vi "Process.vi"(8 "error in":errorcluster, 11 "Instrument":refnum<class "Instrument.lvclass">) -> (0 "error out":errorcluster, 3 "Instrument out":refnum<class "Instrument.lvclass">)   [LabVIEW 2019, in "Instrument.lvlib" / "Instrument.lvclass"]
doc: "---------------------------------------------------------------\nJKI State Machine Objects™\nhttp://jki.net/state-machine-objects/\nCopyright (C) 2005-2015, JKI <info@jki.net>\nALL RIGHTS RESERVED"
uses:
  Instrument.lvclass
  C:/Program Files/National Instruments/LabVIEW 2019/vi.lib/JKI/JKI SMO/SMO/SMO.lvclass
  <userlib>/LevyLab/RemoteControl/RemoteControl/Typedefs/Message--Cluster.ctl
  <vilib>/JKI/JKI SMO/SMO/SMO.lvclass/SMO.ctl
  <vilib>/dlg_ctls.llb/Space Constant.vi
  <vilib>/AdvancedString/1D String Array to Delimited String.vi
  <vilib>/JKI/JKI SMO/SMO/Private/ReftoDVR--SMO.vi
  <userlib>/LevyLab/RemoteControl/RemoteControl/RemoteControl.lvclass
  <userlib>/LevyLab/Logger.Error/Logger.Error/Logger.Error.lvclass
  <userlib>/LevyLab/Logger.PGSQL/Logger.PGSQL/Logger.PGSQL.lvclass
  <vilib>/JKI/JKI SMO/SMO/SMO.lvclass
  <userlib>/LevyLab/Debug/Debug.lvlib
panel:
  out "State History":string
  out "Name":string
  out "Command":string
  # "1. Receives & processes commands from RemoteControl process\n2. Logs instrument settings to PGSQL using Logger process"
  # "INSTRUMENT"
  # "INSTRUMENT"
  # "For instructions on how to use the JKI State Machine Objects, examples and video tutorials, visit:\nhttp://jki.net/state-machine-objects/\n\nJKI State Machine Objects™\nhttp://jki.net/state-machine-objects/\nCopyright (C) 2005-2015, JKI <info@jki.net>\nALL RIGHTS RESERVED"
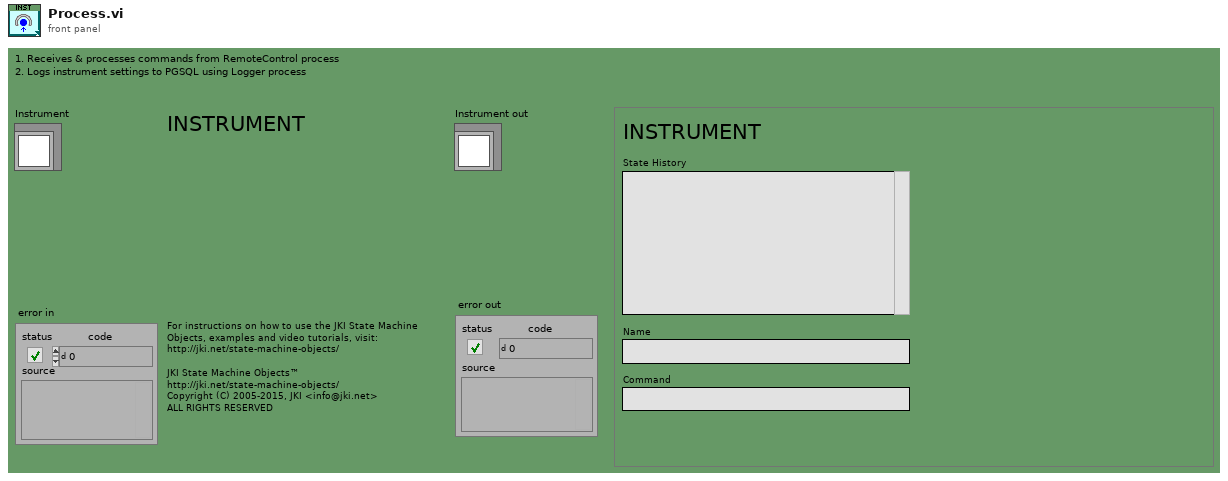
[diagram p1: front panel]
types:
  T1 = enum32{"invalid app kind", "Development System", "Run Time System", "Student Edition", "Embedded LabVIEW", "Evaluation", "Custom"}
  T2 = enum32{"Invalid", "Standard", "Closed", "Hidden", "Minimized", "Maximized"}
  T3 = typedef "RemoteControl.lvlib/RemoteControl.lvclass/Message--Cluster.ctl" = cluster{"Command":string, "Data":variant, "ID":string}
  T4 = typedef "Instrument.lvlib/Instrument.lvclass/Dependencies--Cluster.ctl" = cluster{"API":refnum<class "API.lvclass">, "Configuration":refnum<class "Configuration.lvclass">, "HAL":refnum<class "HAL.lvclass">, "DB-Logger":refnum<class "Logger.PGSQL.lvclass">, "Error-Logger":refnum<class "Logger.Error.lvclass">, "Remote-Control":refnum<class "RemoteControl.lvclass">}
  T5 = cluster{"Core":cluster{"Current VI Reference":refnum<vi>, "Close Panel on Exit?":bool, "Last Error":cluster{"error":errorcluster, "previous state":string, "remaining states":string}, "Shutdown?":bool}, "SelfRef":refnum<class "Instrument.lvclass">, "Dependencies":T4, "Message":T3}
  T6 = typedef "RemoteControl.lvclass/Message--Cluster.ctl" = cluster{"Command":string, "Data":variant, "ID":string}
  T7 = typedef "SMO.lvclass/SMOState --Enum.ctl" = enum16{"unknown", "Created", "Started", "Stopped"}
  T8 = cluster{"Current VI Reference":refnum<vi>, "Close Panel on Exit?":bool, "Last Error":cluster{"error":errorcluster, "previous state":string, "remaining states":string}, "Shutdown?":bool}
  T9 = typedef "Debug.lvlib/Attribute.Debug.lvclass/DebugBehavior.ctl" = enum16{"Normal", "Debug"}
  T10 = typedef "SMO.lvclass/Protected Events.ctl" = cluster{"StopProcesses":refnum<user-event>, "AbortProcesses":refnum<user-event>, "Config Changed":refnum<user-event>, "Dependency":refnum<user-event>}
  T11 = typedef "Instrument.lvlib/Instrument.lvclass/PrivateEvents--Cluster.ctl" = cluster{"MessageToProcess":refnum<user-event>, "LogData":refnum<user-event>, "LogDataMultiline":refnum<user-event>}
  T12 = typedef "RemoteControl.lvlib/RemoteControl.lvclass/PublicEvents--Cluster.ctl" = cluster{"SendMessageFromProcess":refnum<user-event>}
  T13 = typedef "SMO.lvclass/Public Events.ctl" = cluster{"Error":refnum<user-event>, "State":refnum<user-event>, "Reserve State":refnum<user-event>}
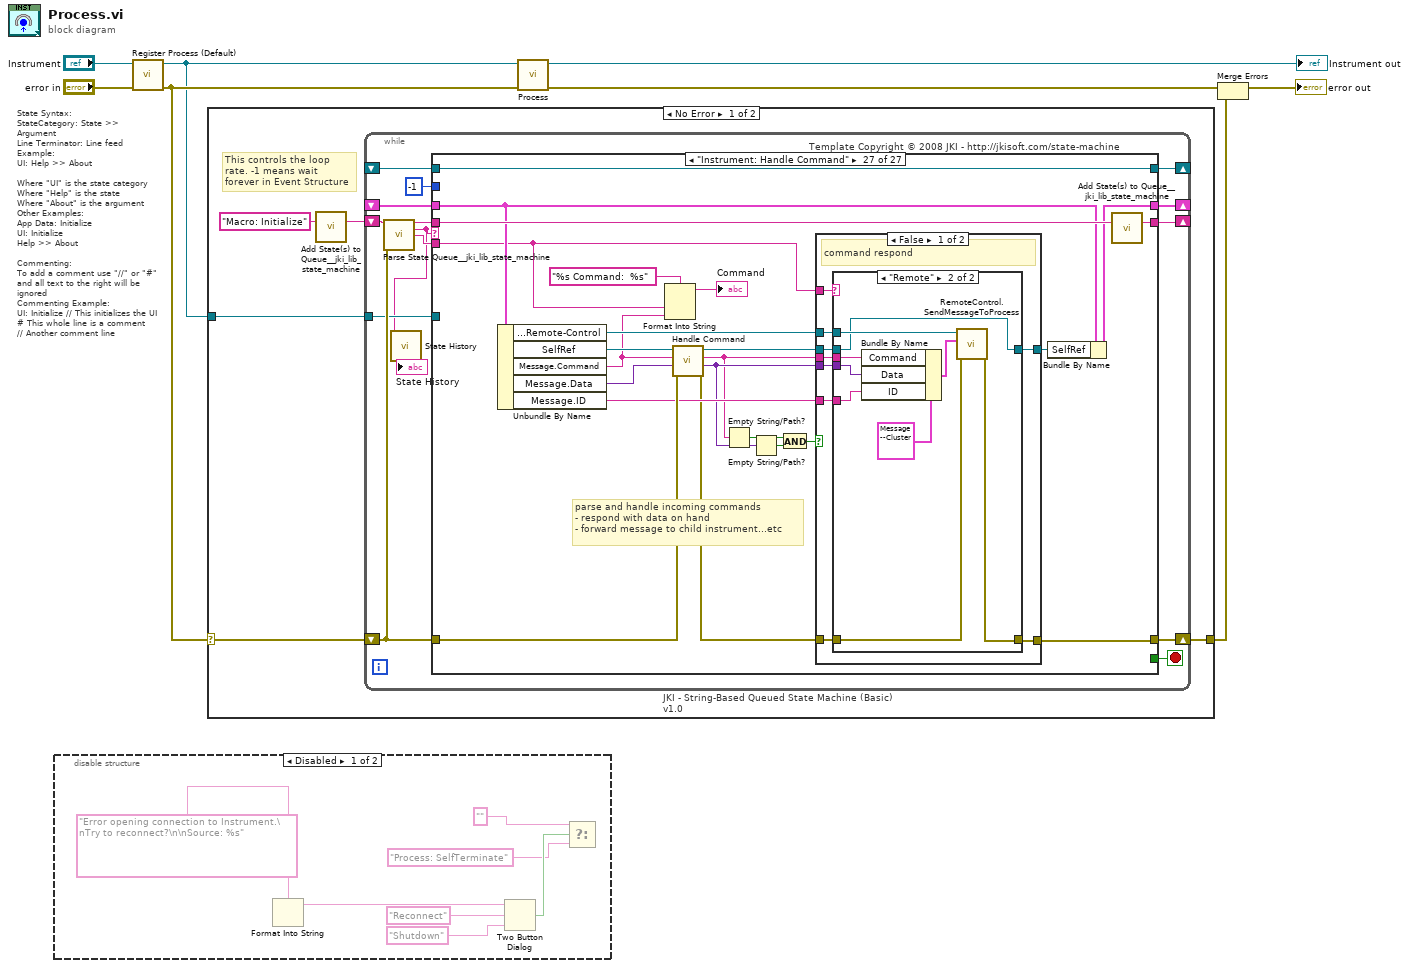
[diagram p0: block diagram]
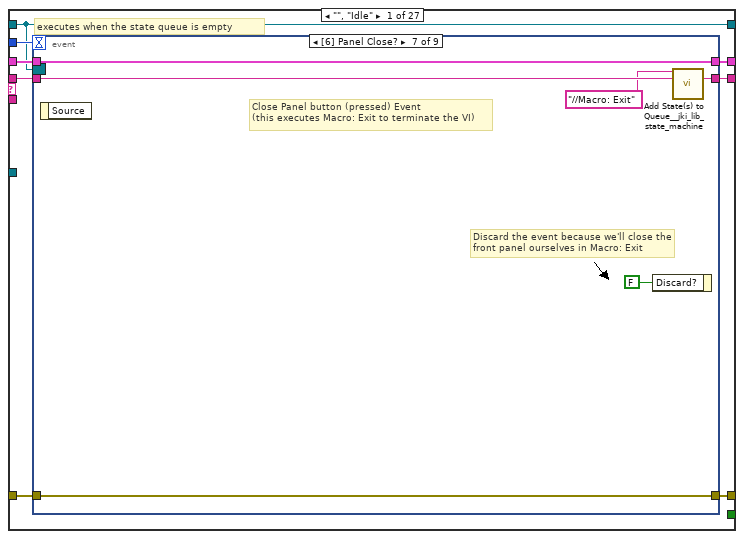
[diagram p3: hidden frame]
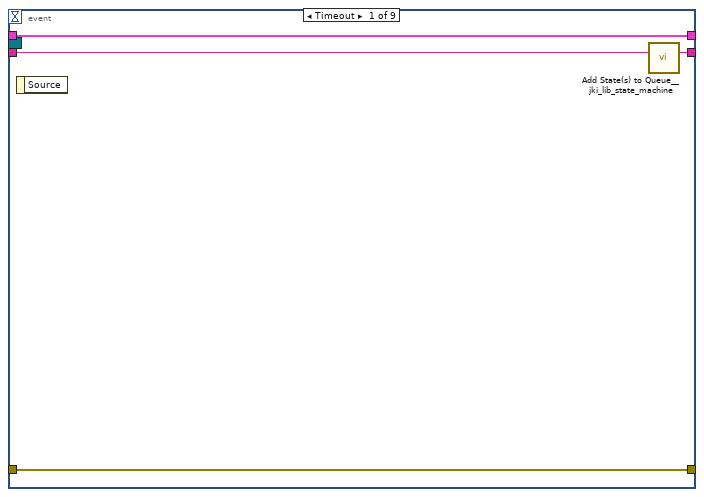
[diagram p4: hidden frame]
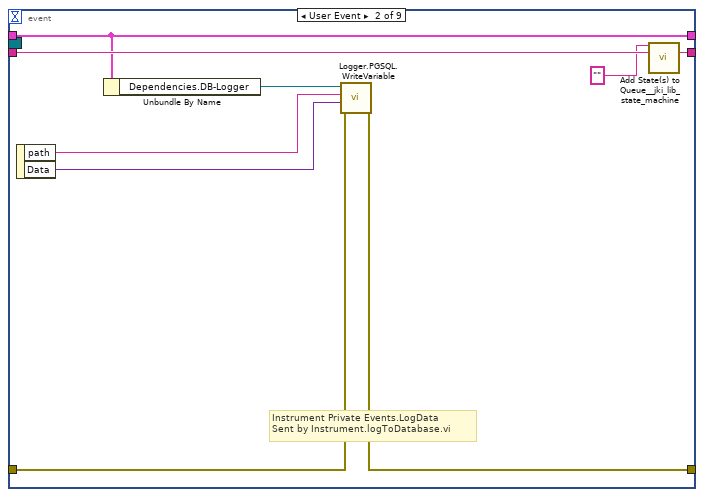
[diagram p5: hidden frame]
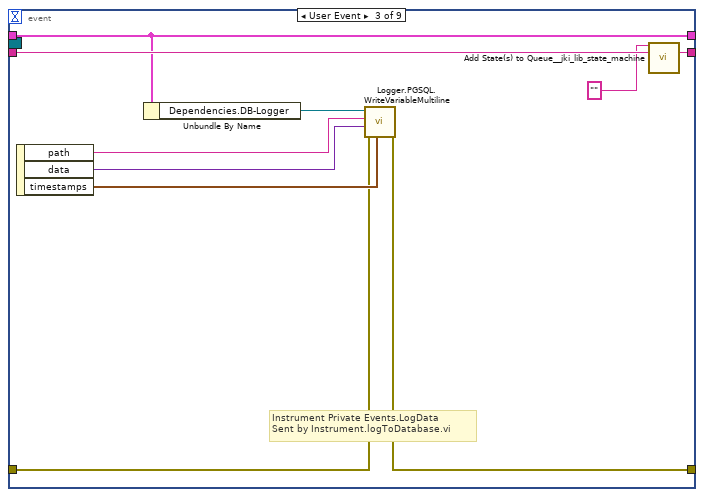
[diagram p6: hidden frame]
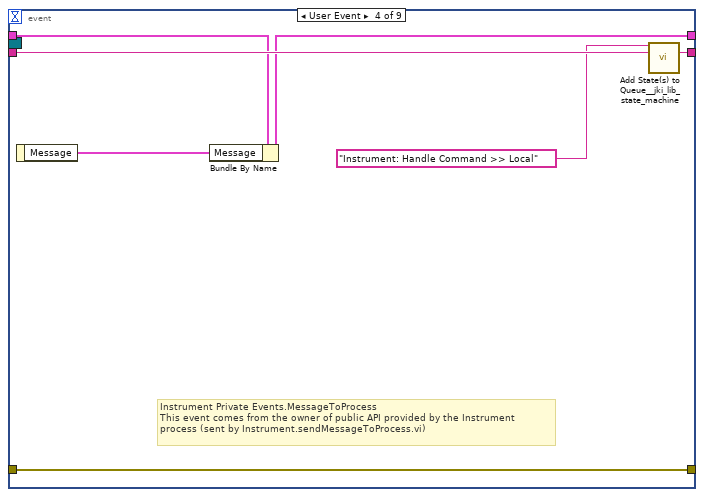
[diagram p7: hidden frame]
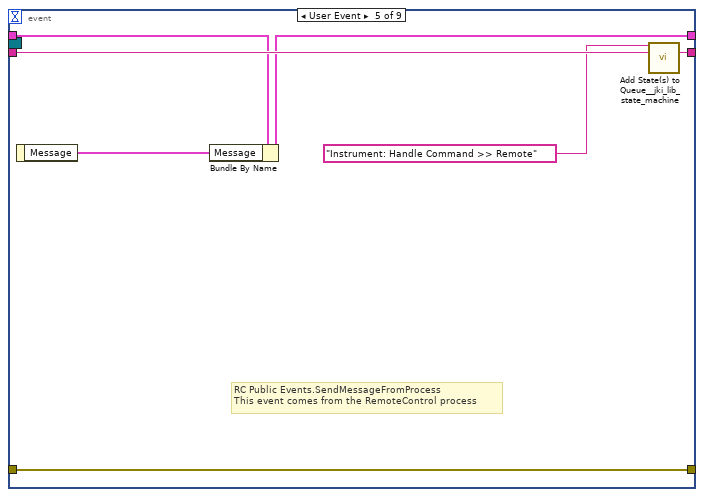
[diagram p8: hidden frame]
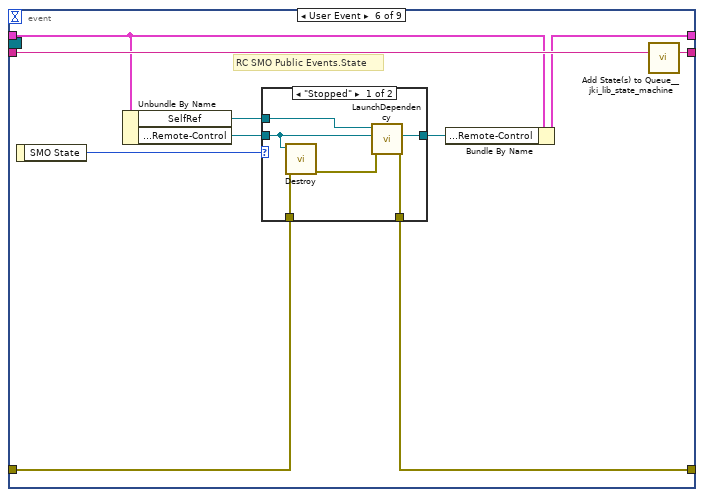
[diagram p9: hidden frame]
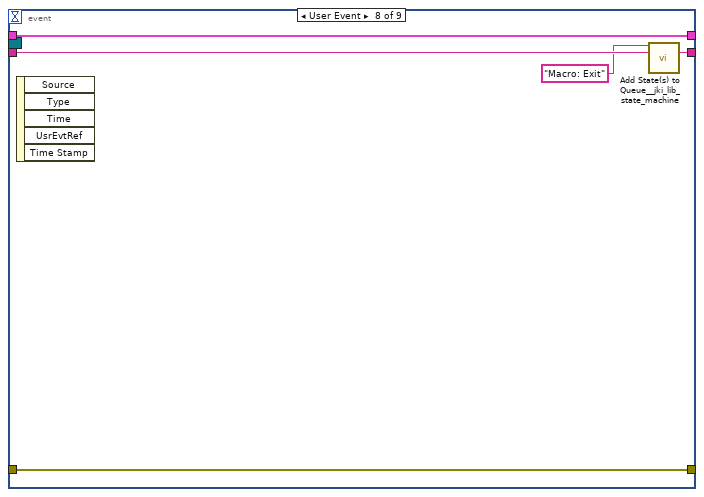
[diagram p11: hidden frame]
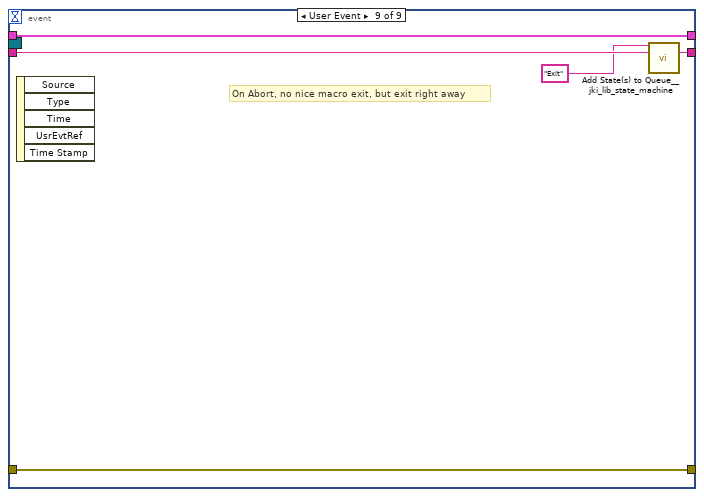
[diagram p12: hidden frame]
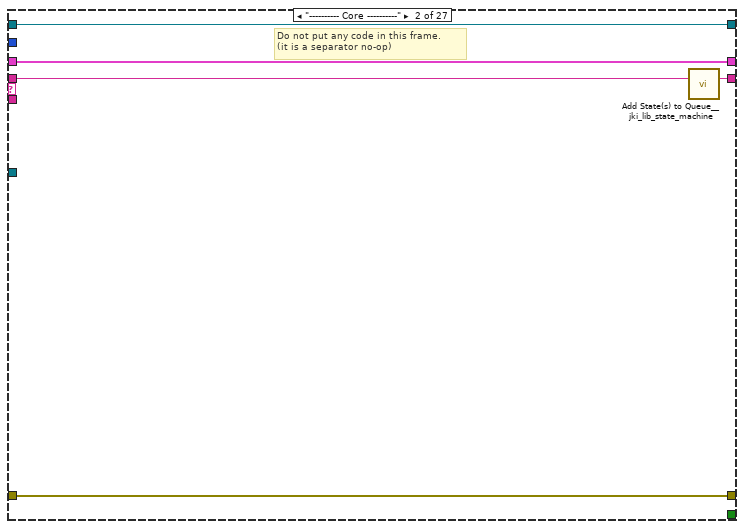
[diagram p13: hidden frame]
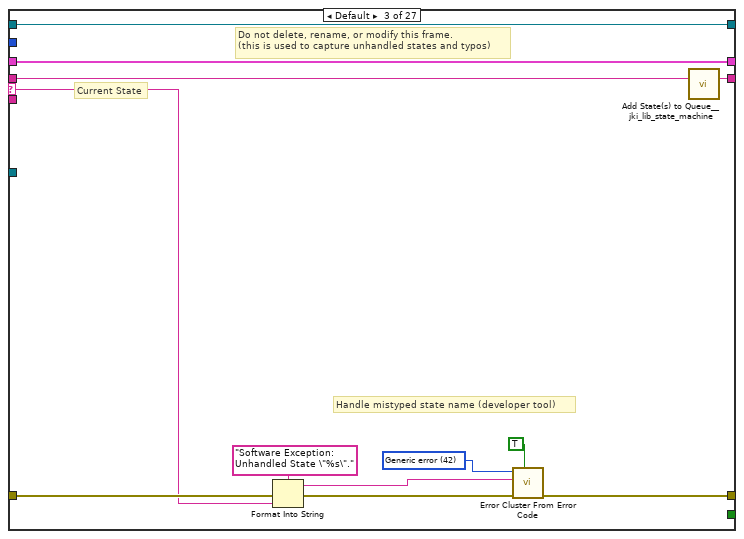
[diagram p14: hidden frame]
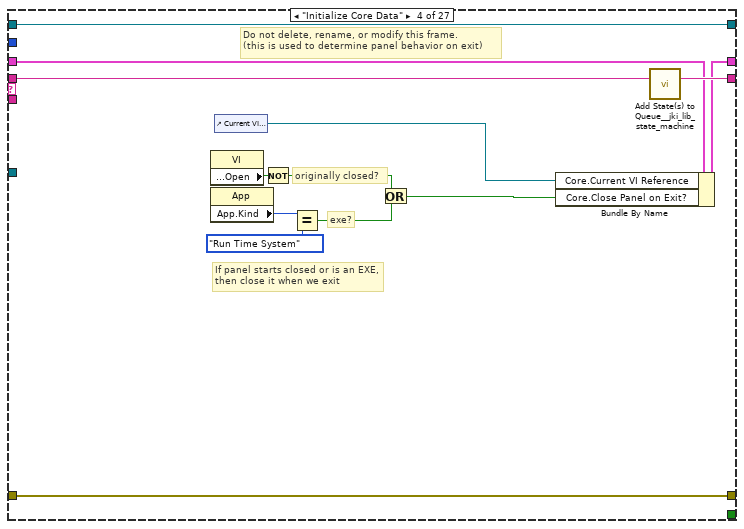
[diagram p15: hidden frame]
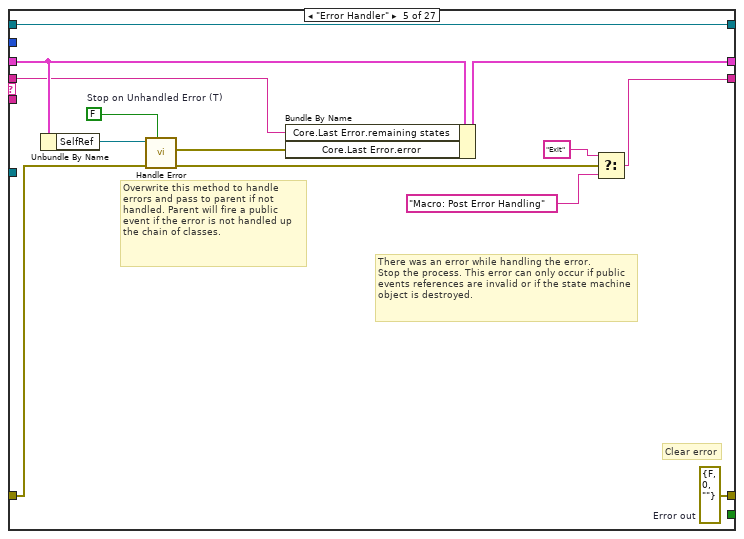
[diagram p16: hidden frame]
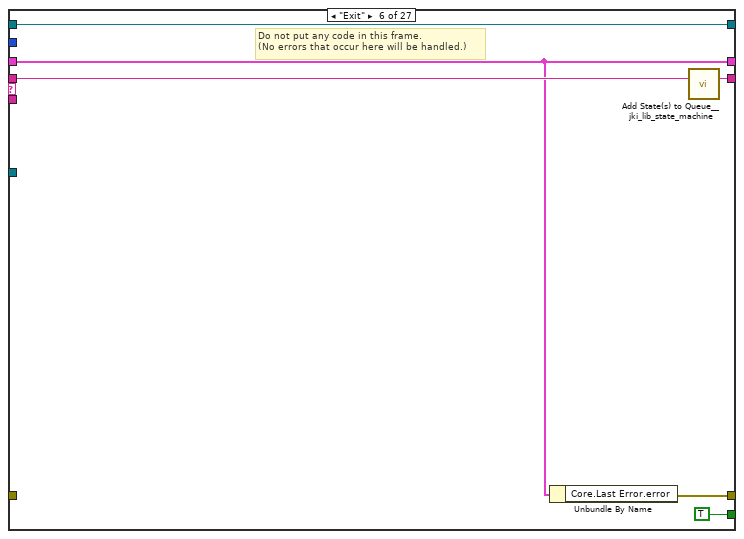
[diagram p17: hidden frame]
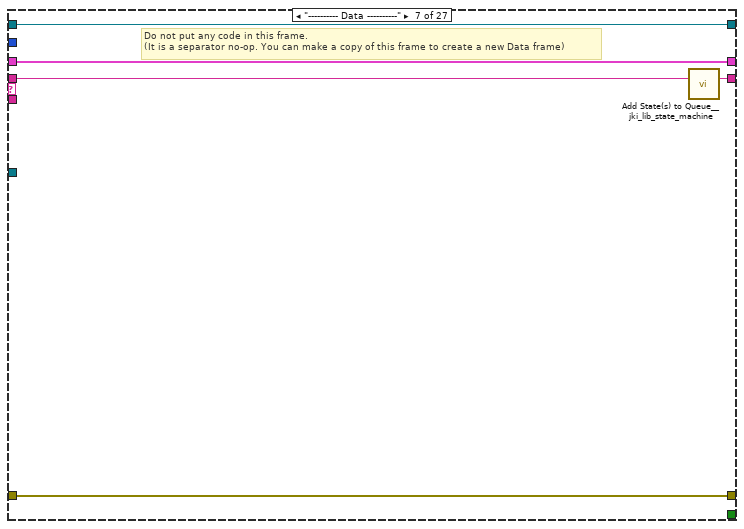
[diagram p18: hidden frame]
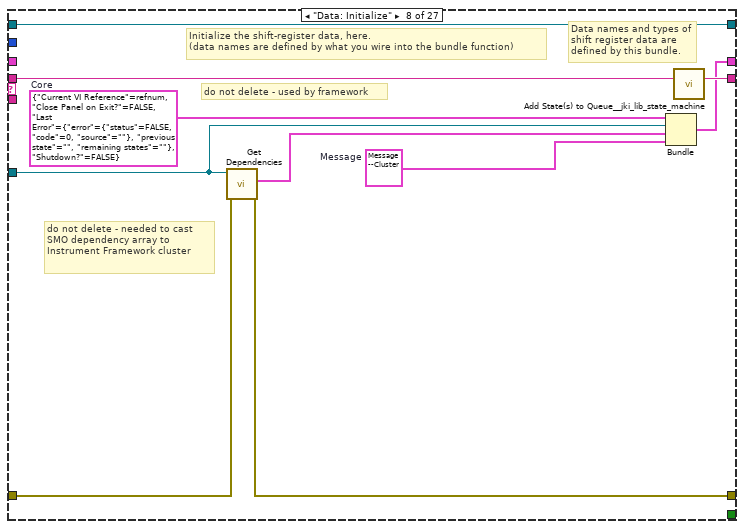
[diagram p19: hidden frame]
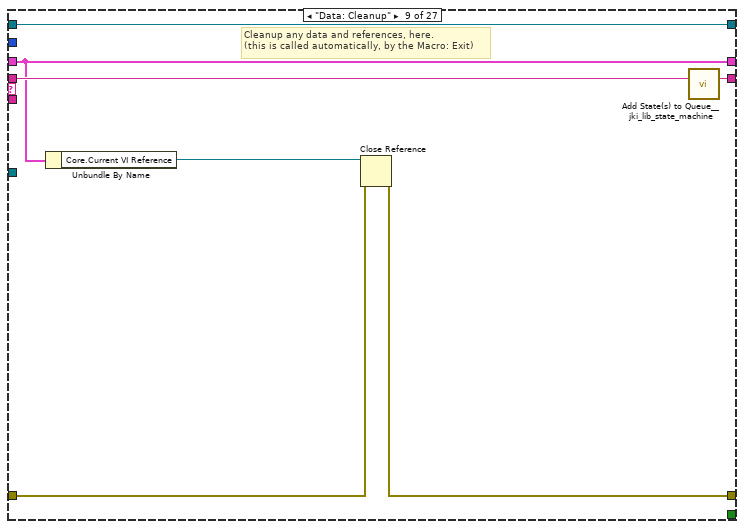
[diagram p20: hidden frame]
diagram:
  # "State Syntax:\nStateCategory: State >> Argument\nLine Terminator: Line feed\nExample:\nUI: Help >> About\n\nWhere \"UI\" is the state category\nWhere \"Help\" is the state\nWhere \"About\" is the argument\nOther Examples:\nApp Data: Initialize\nUI: Initialize\nHelp >> About\n\nCommenting:\nTo add a comment use \"//\" or \"#\" and all text to the right will be ignored\nCommenting Example:\nUI: Initialize // This initializes the UI\n# This whole line is a comment\n// Another comment line"
  n1 = disable-structure shown="Disabled" {
    frame Disabled {
      n2 = Format Into String(format string="Error opening connection to Instrument.\nTry to reconnect?\n\nSource: %s" ("message")) -> (resulting string=w9:string)  [unwired: 3 in, 1 out]
      n3 = Two Button Dialog(message=w9, 1:"Shutdown" ("F button name (\"Cancel\")"), 2:"Reconnect" ("T button name (\"OK\")")) -> (T button?=w13:bool)
      n4 = Select(t="" ("States to Execute"), s=w13, f="Process: SelfTerminate" ("States to Execute")) -> ()  [unwired: 1 out]
    }
    frame Enabled {
    }
  }
  n5 = call <vilib>:"Register Process (Default).vi"("error in (no error)"="error in", "SMO"="Instrument") -> ("error out"=w5:errorcluster, "SelfRef"=w4:refnum<class "Instrument.lvclass">)  [unwired: 8 in]
  n6 = case shown="No Error" w5 {
    selector: w5 -> [w17 w448]
    tunnel: w4 -> [w18 _]
    tunnel: [w16 w448] -> w1
    frame No Error {
      # "This controls the loop rate. -1 means wait forever in Event Structure"
      n7 = call <vilib>:"Add State(s) to Queue__jki_lib_state_machine.vi"("State(s) in (\"\")"="Macro: Initialize") -> ("States Out"=w20:string)  [unwired: 14 in]
      n8 = while "JKI - String-Based Queued State Machine (Basic) v1.0" {
        shift-right: [w29] -> _
        shift-left: _ -> [w28]
        shift-right: [w32] -> w16
        shift-left: w17 -> [w26]
        shift-right: [w31] -> _
        shift-left: w20 -> [w33]
        tunnel: w18 -> [w23]
        shift-right: [w25] -> _
        shift-left: _ -> [w24]
        stop <- w30 stop-if-true
        # "Template Copyright © 2008 JKI - http://jkisoft.com/state-machine"
        n9 = call <vilib>:"Parse State Queue__jki_lib_state_machine.vi"("State Queue"=w33, "Error In (no error)"=w26) -> ("Remaining States"=w35:string, "Current State"=w22:string, "Arguments"=w34:string)  [unwired: 11 in]
        n10 = call "State History.vi"("Current State"=w22) -> ("History"=→"State History":string)  [unwired: 10 in]
        n11 = case shown="\"Instrument: Handle Command\"" w22 {
          selector: w22 -> [_ _ w121 _ _ _ _ _ _ _ _ _ _ _ _ _ _ _ _ _ _ _ _ _ _ _ _]
          tunnel: w35 -> [w43 w119 w125 w144 w146 w163 w168 w178 w185 w190 w200 w207 w223 w259 w264 w273 w289 w293 w320 w330 w341 w350 w355 w386 w392 w397 w420]
          tunnel: w34 -> [_ _ _ _ _ _ _ _ _ _ _ w201 w217 w253 _ _ _ _ _ _ _ _ _ _ _ _ w400]
          tunnel: w28 -> [w41 w116 w123 w135 w155 w159 w165 _ w180 w187 w197 w205 w219 w256 w261 w267 w275 w296 w309 w327 w338 w345 w352 w384 w390 w395 w413]
          tunnel: [w40 w117 w127 w141 w156 w158 w166 w170 w181 w188 w191 w202 w220 w252 w262 w266 w287 w300 w308 w328 w332 w342 w353 w382 w388 w393 w405] -> w32
          tunnel: w26 -> [w39 w117 w126 w141 w147 _ w166 w171 w182 w188 w194 w203 w221 w252 w262 w266 w287 w300 w307 w328 w333 w343 w353 w380 w388 w393 w416]
          tunnel: [w42 w118 w124 w143 w151 w162 w167 w177 w184 w189 w199 w206 w222 w258 w263 w272 w288 w294 w319 w329 w340 w349 w354 w385 w391 w396 w419] -> w31
          tunnel: [_ _ _ _ _ TRUE _ _ _ _ _ _ _ _ _ _ _ _ _ _ _ _ _ _ _ _ _] -> w30
          tunnel: [w38 w116 w123 w142 w154 w159 w165 w169 w180 w187 w197 w205 w219 w256 w261 w267 w276 w297 w310 w327 w338 w344 w352 w384 w390 w395 w412] -> w29
          tunnel: -1 ("Timeout") -> [w37 _ _ _ _ _ _ _ _ _ _ _ _ _ _ _ _ _ _ _ _ _ _ _ _ _ _]
          tunnel: [w36 w115 w120 w132 w157 w160 w164 w176 w179 w186 w198 w204 w216 w257 w260 w271 w282 w301 w318 w326 w339 w348 w351 w383 w389 w394 w418] -> w25
          tunnel: w24 -> [w36 w115 w120 w132 w157 w160 w164 w176 w179 w186 w198 w204 w216 w257 w260 w271 w282 w301 w318 w326 w339 w348 w351 _ w389 w394 w418]
          tunnel: w23 -> [_ _ _ _ _ _ _ w172 _ _ _ _ _ _ _ _ _ _ _ _ _ _ _ _ _ _ _]
          frame "", "Idle" {
            # "executes when the state queue is empty"
            n12 = event shown="[6] Panel Close?" {
              selector: w36 -> [_ _ _ _ _ _ _ _ _]
              dyn-events: _ -> [_ _ _ _ _ _ _ _ _]
              timeout: w37 -> [_ _ _ _ _ _ _ _ _]
              tunnel: w43 -> [w47 w56 w66 w73 w80 w90 w104 w109 w114]
              tunnel: [w46 w55 w65 w72 w79 w89 w103 w108 w113] -> w42
              tunnel: w41 -> [w44 w48 w57 w70 w77 w86 w101 w106 w111]
              tunnel: [w45 w50 w59 w71 w78 w83 w102 w107 w112] -> w40
              tunnel: w39 -> [w45 w49 w58 w71 w78 w84 w102 w107 w112]
              tunnel: [w44 w48 w57 w69 w76 w85 w101 w106 w111] -> w38
              event Timeout {
                n13 = event-data() -> ()  [unwired: 1 in, 1 out]
                n14 = call <vilib>:"Add State(s) to Queue__jki_lib_state_machine.vi"("State(s) in (\"\")"=w47) -> ("States Out"=w46:string)  [unwired: 14 in]
              }
              event User Event {
                # "Instrument Private Events.LogData\nSent by Instrument.logToDatabase.vi"
                n15 = event-data() -> ("path"=w51:string, "Data"=w52:variant)  [unwired: 1 in]
                n16 = Unbundle By Name(w48) -> ("Dependencies.DB-Logger"=w53:refnum<class "Logger.PGSQL.lvclass">)
                n17 = call <userlib>:"Logger.PGSQL.WriteVariable.vi"("error in (no error)"=w49, "Data"=w52, "Address"=w51, "Logger"=w53) -> ("error out"=w50:errorcluster)  [unwired: 6 in, 1 out]
                n18 = call <vilib>:"Add State(s) to Queue__jki_lib_state_machine.vi"("State(s) in Front (\"\")"="" ("State(s) in Front (\"\")"), "State(s) in (\"\")"=w56) -> ("States Out"=w55:string)  [unwired: 13 in]
              }
              event User Event {
                # "Instrument Private Events.LogData\nSent by Instrument.logToDatabase.vi"
                n19 = event-data() -> ("path"=w62:string, "data"=w61:variant, "timestamps"=w60:timestamp[])  [unwired: 1 in]
                n20 = Unbundle By Name(w57) -> ("Dependencies.DB-Logger"=w63:refnum<class "Logger.PGSQL.lvclass">)
                n21 = call <userlib>:"Logger.PGSQL.WriteVariableMultiline.vi"("Timestamps"=w60, "error in (no error)"=w58, "Data"=w61, "Address"=w62, "Logger"=w63) -> ("error out"=w59:errorcluster)  [unwired: 5 in, 1 out]
                n22 = call <vilib>:"Add State(s) to Queue__jki_lib_state_machine.vi"("State(s) in Front (\"\")"="" ("State(s) in Front (\"\")"), "State(s) in (\"\")"=w66) -> ("States Out"=w65:string)  [unwired: 13 in]
              }
              event User Event {
                # "Instrument Private Events.MessageToProcess\nThis event comes from the owner of public API provided by the Instrument\nprocess (sent by Instrument.sendMessageToProcess.vi)"
                n23 = event-data() -> ("Message"=w68:T3)  [unwired: 1 in]
                n24 = Bundle By Name(cluster=w70, "Message"=w68) -> (w69:T5)
                n25 = call <vilib>:"Add State(s) to Queue__jki_lib_state_machine.vi"("State(s) in Front (\"\")"="Instrument: Handle Command >> Local" ("State(s) in Front (\"\")"), "State(s) in (\"\")"=w73) -> ("States Out"=w72:string)  [unwired: 13 in]
              }
              event User Event {
                # "RC Public Events.SendMessageFromProcess\nThis event comes from the RemoteControl process"
                n26 = event-data() -> ("Message"=w75:T6)  [unwired: 1 in]
                n27 = Bundle By Name(cluster=w77, "Message"=w75) -> (w76:T5)
                n28 = call <vilib>:"Add State(s) to Queue__jki_lib_state_machine.vi"("State(s) in Front (\"\")"="Instrument: Handle Command >> Remote" ("State(s) in Front (\"\")"), "State(s) in (\"\")"=w80) -> ("States Out"=w79:string)  [unwired: 13 in]
              }
              event User Event {
                # "RC SMO Public Events.State"
                n29 = event-data() -> ("SMO State"=w81:T7)  [unwired: 1 in]
                n30 = Unbundle By Name(w86) -> ("SelfRef"=w82:refnum<class "Instrument.lvclass">, "Dependencies.Remote-Control"=w88:refnum<class "RemoteControl.lvclass">)
                n31 = case shown="\"Stopped\"" w81 {
                  tunnel: w88 -> [w91 w98]
                  tunnel: [w96 w98] -> w87
                  tunnel: w84 -> [w93 w97]
                  tunnel: [w95 w97] -> w83
                  tunnel: w82 -> [w94 _]
                  frame "Stopped" {
                    n32 = call <vilib>:"Destroy.vi"("error in (no error)"=w93, "SMO"=w91) -> ("error out"=w92:errorcluster)  [unwired: 9 in]
                    n33 = call <vilib>:"LaunchDependency.vi"("error in (no error)"=w92, "Dependency Type"=w91, "SMO in"=w94) -> ("error out"=w95:errorcluster, "Dependency Reference"=w96:refnum<class "RemoteControl.lvclass">)  [unwired: 5 in, 2 out]
                  }
                  frame Default {
                  }
                }
                n34 = Bundle By Name(cluster=w86, "Dependencies.Remote-Control"=w87) -> (w85:T5)
                n35 = call <vilib>:"Add State(s) to Queue__jki_lib_state_machine.vi"("State(s) in (\"\")"=w90) -> ("States Out"=w89:string)  [unwired: 14 in]
              }
              event Panel Close? {
                # "Discard the event because we'll close the front panel ourselves in Macro: Exit"
                # "Close Panel button (pressed) Event\n(this executes Macro: Exit to terminate the VI)"
                n36 = event-data() -> ()  [unwired: 1 in, 1 out]
                n37 = event-data("Discard?"=FALSE) -> ()  [unwired: 1 in, 1 out]
                n38 = call <vilib>:"Add State(s) to Queue__jki_lib_state_machine.vi"("State(s) in Front (\"\")"="//Macro: Exit", "State(s) in (\"\")"=w104) -> ("States Out"=w103:string)  [unwired: 13 in]
              }
              event User Event {
                n39 = event-data() -> ()  [unwired: 1 in, 5 out]
                n40 = call <vilib>:"Add State(s) to Queue__jki_lib_state_machine.vi"("State(s) in Front (\"\")"="Macro: Exit", "State(s) in (\"\")"=w109) -> ("States Out"=w108:string)  [unwired: 13 in]
              }
              event User Event {
                # "On Abort, no nice macro exit, but exit right away"
                n41 = event-data() -> ()  [unwired: 1 in, 5 out]
                n42 = call <vilib>:"Add State(s) to Queue__jki_lib_state_machine.vi"("State(s) in Front (\"\")"="Exit", "State(s) in (\"\")"=w114) -> ("States Out"=w113:string)  [unwired: 13 in]
              }
            }
          }
          frame "---------- Core ----------" {
            # "Do not put any code in this frame.\n(it is a separator no-op)"
            n43 = call <vilib>:"Add State(s) to Queue__jki_lib_state_machine.vi"("State(s) in (\"\")"=w119) -> ("States Out"=w118:string)  [unwired: 14 in]
          }
          frame Default {
            w130 = 42 items=["No error", "Argument error", "Memory is full", "Out of zone", "End of file", "File already open", "Generic file I/O error", "File not found", "File permission error", "Disk is full", "Duplicate path", "Too many files open", "System feature not enabled", "Resource file not found", "Cannot add resource", "Resource not found", "Image not found", "Image memory error", "Pen does not exist", "Config type invalid", "Config token not found", "Config parse error", "Config memory error", "Bad external code format", "Bad external code offset", "External code not present", "Null window", "Destroy window error", "Null menu", "Print aborted", "Bad print record", "Print driver error", "Windows error during printing", "Memory error during printing", "Print dialog error", "Generic print error", "Invalid device refnum", "Device not found", "Device parameter error", "Device unit error", "Cannot open device", "Device call aborted", "Generic error", "Cancelled by user", "Object ID too low", "Object ID too high", "Object not in heap", "Unknown heap", "Unknown object (invalid DefProc)", "Unknown object (DefProc not in table)", "Message out of range", "Invalid (null) method", "Unknown message", "Manager call not supported", "Bad address", "Network operation in progress", "Network operation timed out", "Connection is busy", "Network attribute not supported", "Network error", "Address in use", "System out of memory", "Connection aborted", "Connection refused", "Not connected", "Already connected", "Connection closed", "Initialization error (interapplication manager)", "Bad occurrence", "Wait on unbound occurrence handler", "Occurrence queue overflow", "Datalog type conflict", "Unused", "Unrecognized type (interapplication manager)", "Memory corrupt", "Failed to make temporary DLL", "Old CIN version", "Drag socket not found", "Failed to load drop-object", "Failed to register OLE object", "Failed to release OLE object", "Format specifier type mismatch", "Unknown format specifier", "Too few format specifiers", "Too many format specifiers", "Scan failed", "Newer CIN version", "Error converting to variant", "Runtime menu error", "Password tampered", "Variant attribute not found", "Incompatible variant data type", "Event data is not available", "Event Store is not present", "Occurrence is not found", "Event Queue is not created", "Event info is not available", "Refnum passed is NULL", "Error retrieving Class GUID", "Error retrieving CoClass GUID", "Error retrieving TypeLib GUID.", "Bad built application magic bytes.", "Specific driver is different from the specific driver associated with the Logical Name.", "There is no session opened to the class driver.", "Max Error", "MAX - Error with config objects", "MAX - Error loading configuration", "MAX - Group not supported"]
            # "Current State"
            # "Do not delete, rename, or modify this frame.\n(this is used to capture unhandled states and typos)"
            # "Handle mistyped state name (developer tool)"
            n44 = Format Into String(format string="Software Exception: Unhandled State \"%s\"." ("message"), error in=w126, w121) -> (resulting string=w129:string, error out=w128:errorcluster)  [unwired: 1 in]
            n45 = call <vilib>:"Error Cluster From Error Code.vi"("show call chain? (False)"=TRUE, "error in (no error)"=w128, "error message (\"\")"=w129, "error code (0)"=w130) -> ("error out"=w127:errorcluster)  [unwired: 5 in]
            n46 = call <vilib>:"Add State(s) to Queue__jki_lib_state_machine.vi"("State(s) in (\"\")"=w125) -> ("States Out"=w124:string)  [unwired: 14 in]
          }
          frame "Initialize Core Data" {
            # "Do not delete, rename, or modify this frame.\n(this is used to determine panel behavior on exit)"
            # "originally closed?"
            # "exe?"
            # "If panel starts closed or is an EXE, then close it when we exit"
            n47 = property class="VI"() -> ("Front Panel.Open"=w140:bool)  [unwired: 2 in, 2 out]
            n48 = property class="App"() -> ("App.Kind"=w139:T1)  [unwired: 2 in, 2 out]
            n49 = control-ref of="Current VI Reference"() -> (w133:refnum<vi>)
            n50 = Not(x=w140) -> (.not. x?=w137:bool)
            n51 = Equal?(x=w139, y=T1."Run Time System" ("Application:Kind")) -> (x = y?=w136:bool)
            n52 = Or(x=w137, y=w136) -> (x .or. y?=w134:bool)
            n53 = Bundle By Name(cluster=w135, "Core.Current VI Reference"=w133, "Core.Close Panel on Exit?"=w134) -> (w142:T5)
            n54 = call <vilib>:"Add State(s) to Queue__jki_lib_state_machine.vi"("State(s) in (\"\")"=w144) -> ("States Out"=w143:string)  [unwired: 14 in]
          }
          frame "Error Handler" {
            w152 = FALSE  # Stop on Unhandled Error (T)
            w156 = errorcluster {"status"=FALSE, "code"=0, "source"=""}  # Error out
            # "Clear error"
            # "There was an error while handling the error.\nStop the process. This error can only occur if public events references are invalid or if the state machine object is destroyed."
            # "Overwrite this method to handle errors and pass to parent if not handled. Parent will fire a public event if the error is not handled up the chain of classes."
            n55 = Unbundle By Name(w155) -> ("SelfRef"=w148:refnum<class "Instrument.lvclass">)
            n56 = call-dynamic "Handle Error.vi"("Stop on Unhandled Error (T)"=w152, "error in"=w147, "SMO"=w148) -> ("handling error"=w149:errorcluster, "Unhandled error"=w150:errorcluster)  [unwired: 6 in, 1 out]
            n57 = Bundle By Name(cluster=w155, "Core.Last Error.remaining states"=w146, "Core.Last Error.error"=w150) -> (w154:T5)
            n58 = Select(t="Exit", s=w149, f="Macro: Post Error Handling" ("State")) -> (s? t:f=w151:string)
          }
          frame "Exit" {
            # "Do not put any code in this frame.\n(No errors that occur here will be handled.)"
            n59 = Unbundle By Name(w159) -> ("Core.Last Error.error"=w158:errorcluster)
            n60 = call <vilib>:"Add State(s) to Queue__jki_lib_state_machine.vi"("State(s) in (\"\")"=w163) -> ("States Out"=w162:string)  [unwired: 14 in]
          }
          frame "---------- Data ----------" {
            # "Do not put any code in this frame.\n(It is a separator no-op. You can make a copy of this frame to create a new Data frame)"
            n61 = call <vilib>:"Add State(s) to Queue__jki_lib_state_machine.vi"("State(s) in (\"\")"=w168) -> ("States Out"=w167:string)  [unwired: 14 in]
          }
          frame "Data: Initialize" {
            w174 = T3 {"Command"="", "Data"=variant(string ""), "ID"=""}  # Message
            w175 = T8 {"Current VI Reference"=refnum, "Close Panel on Exit?"=FALSE, "Last Error"={"error"={"status"=FALSE, "code"=0, "source"=""}, "previous state"="", "remaining states"=""}, "Shutdown?"=FALSE}  # Core
            # "do not delete - needed to cast SMO dependency array to Instrument Framework cluster"
            # "do not delete - used by framework"
            # "Data names and types of shift register data are defined by this bundle."
            # "Initialize the shift-register data, here.\n(data names are defined by what you wire into the bundle function)"
            n62 = call "Get Dependencies.vi"("error in (no error)"=w171, "Instrument in"=w172) -> ("error out"=w170:errorcluster, "Dependencies"=w173:T4)  [unwired: 7 in, 1 out]
            n63 = Bundle("Core"=w175, "SelfRef"=w172, "Dependencies"=w173, "Message"=w174) -> (w169:T5)  [unwired: 1 in]
            n64 = call <vilib>:"Add State(s) to Queue__jki_lib_state_machine.vi"("State(s) in (\"\")"=w178) -> ("States Out"=w177:string)  [unwired: 14 in]
          }
          frame "Data: Cleanup" {
            # "Cleanup any data and references, here.\n(this is called automatically, by the Macro: Exit)"
            n65 = Unbundle By Name(w180) -> ("Core.Current VI Reference"=w183:refnum<vi>)
            n66 = Close Reference(reference=w183, error in (no error)=w182) -> (error out=w181:errorcluster)
            n67 = call <vilib>:"Add State(s) to Queue__jki_lib_state_machine.vi"("State(s) in (\"\")"=w185) -> ("States Out"=w184:string)  [unwired: 14 in]
          }
          frame "---------- UI ----------" {
            # "Do not put any code in this frame.\n(It is a separator no-op. You can make a copy of this frame to create a new UI frame)"
            n68 = call <vilib>:"Add State(s) to Queue__jki_lib_state_machine.vi"("State(s) in (\"\")"=w190) -> ("States Out"=w189:string)  [unwired: 14 in]
          }
          frame "UI: Initialize" {
            # "Initialize the User Interface, here.\n(this is called automatically, by the Macro: Init)"
            n69 = Unbundle By Name(w197) -> ("SelfRef"=w196:refnum<class "Instrument.lvclass">)
            n70 = call <vilib>:"GetName.vi"("error in (no error)"=w194, "SMO"=w196) -> ("error out"=w192:errorcluster, "Name"=→"Name":string)  [unwired: 6 in, 2 out]
            n71 = call <userlib>:"Fit VI window to Largest Dec__ogtk.vi"("error in (no error)"=w192, "border spacing (2 px)"=0) -> ("error out"=w191:errorcluster)  [unwired: 4 in, 1 out]
            n72 = call <vilib>:"Add State(s) to Queue__jki_lib_state_machine.vi"("State(s) in (\"\")"=w200) -> ("States Out"=w199:string)  [unwired: 14 in]
          }
          frame "UI: Cursor Set" {
            # "Argument"
            # "Initialize the User Interface, here.\n(this is called automatically, by the Macro: Init)"
            n73 = disable-structure shown="Default" {
              disable-tunnel: w203 -> [w208 w211]
              disable-tunnel: [w208 w210] -> w202
              disable-tunnel: w201 -> [_ w209]
              frame condition #0 {
              }
              frame condition #1 (active) {
                n74 = case shown="\"Busy\"" w209 {
                  tunnel: w211 -> [w213 w215]
                  tunnel: [w212 w214] -> w210
                  frame "Idle", Default {
                    n75 = call <vilib>:"Unset Busy.vi"("error in (no error)"=w213) -> ("error out"=w212:errorcluster)  [unwired: 10 in]
                  }
                  frame "Busy" {
                    n76 = call <vilib>:"Set Busy.vi"("error in (no error)"=w215) -> ("error out"=w214:errorcluster)  [unwired: 9 in, 1 out]
                  }
                }
              }
            }
            n77 = call <vilib>:"Add State(s) to Queue__jki_lib_state_machine.vi"("State(s) in (\"\")"=w207) -> ("States Out"=w206:string)  [unwired: 14 in]
          }
          frame "UI: Front Panel State" {
            # "Argument"
            # "Set Front Panel Open or Closed\n(Usage: \"UI: Front Panel State >> Open|Close\")"
            n78 = Unbundle By Name(w219) -> ("Core.Current VI Reference"=w218:refnum<vi>)
            n79 = disable-structure shown="Default" {
              disable-tunnel: w221 -> [w227 w250]
              disable-tunnel: [w226 w250] -> w220
              disable-tunnel: w218 -> [w225 _]
              disable-tunnel: w217 -> [w224 _]
              frame condition #0 (active) {
                n80 = case shown="\"Close\"" w224 {
                  tunnel: w227 -> [w231 w244]
                  tunnel: [w233 w245] -> w226
                  tunnel: w225 -> [w232 w242]
                  frame "Open", Default {
                    n81 = property class="VI"(reference=w232, error in=w231) -> (reference out=w229:refnum<vi>, error out=w230:errorcluster, "FP.State"=w228:T2)
                    n82 = case shown="Default" w228 {
                      tunnel: [w236 w239] -> w233
                      tunnel: w230 -> [w235 w239]
                      tunnel: w229 -> [w234 _]
                      frame "Closed" {
                        n83 = invoke class="VI" method="FP.Open"(reference=w234, error in=w235, "Activate"=TRUE, "State"=T2."Standard") -> (error out=w236:errorcluster)  [unwired: 1 in, 4 out]
                      }
                      frame Default {
                      }
                    }
                  }
                  frame "Close" {
                    n84 = property class="VI"(reference=w242, error in=w244) -> (reference out=w241:refnum<vi>, error out=w243:errorcluster, "FP.State"=w240:T2)
                    n85 = case shown="Default" w240 {
                      tunnel: [w246 w249] -> w245
                      tunnel: w243 -> [w246 w248]
                      tunnel: w241 -> [_ w247]
                      frame "Invalid", "Closed" {
                      }
                      frame Default {
                        n86 = invoke class="VI" method="FP.Close"(reference=w247, error in=w248) -> (error out=w249:errorcluster)  [unwired: 1 in, 2 out]
                      }
                    }
                  }
                }
              }
              frame condition #1 {
              }
            }
            n87 = call <vilib>:"Add State(s) to Queue__jki_lib_state_machine.vi"("State(s) in (\"\")"=w223) -> ("States Out"=w222:string)  [unwired: 14 in]
          }
          frame "UI: Wait" {
            n88 = Scan From String(format string="%d", input string=w253, default 1=u32 0 ("default value 1")) -> (output 1=w251:u32)  [unwired: 2 in, 3 out]
            n89 = Wait (ms)(milliseconds to wait=w251) -> ()  [unwired: 1 out]
            n90 = call <vilib>:"Add State(s) to Queue__jki_lib_state_machine.vi"("State(s) in (\"\")"=w259) -> ("States Out"=w258:string)  [unwired: 14 in]
          }
          frame "---------- Macro ----------" {
            # "Do not put any code in this frame.\n(It is a separator no-op. You can make a copy of this frame to create a new Macro frame)"
            n91 = call <vilib>:"Add State(s) to Queue__jki_lib_state_machine.vi"("State(s) in (\"\")"=w264) -> ("States Out"=w263:string)  [unwired: 14 in]
          }
          frame "Macro: Initialize" {
            # "Initialization Macro\n(This is called once, when the VI starts)"
            n92 = call <vilib>:"Add State(s) to Queue__jki_lib_state_machine.vi"("State(s) in Front (\"\")"="Data: Initialize\nInitialize Core Data\nEvents: Register", "State(s) in (\"\")"="Process: Sync", "State(s) at Back (\"\")"="UI: Initialize\nUI: Front Panel State >> Close\nMacro: Debug") -> ("States Out"=w269:string)  [unwired: 12 in]
            n93 = call <vilib>:"Add State(s) to Queue__jki_lib_state_machine.vi"("State(s) in Front (\"\")"=w269, "State(s) in (\"\")"=w273) -> ("States Out"=w272:string)  [unwired: 13 in]
          }
          frame "Macro: Exit" {
            # "Exit Macro\n(This is called once, when the VI exits)"
            n94 = Unbundle By Name(w275) -> ("Core.Close Panel on Exit?"=w286:bool)
            n95 = Select(t="UI: Front Panel State >> Close", s=w286, f="") -> (s? t:f=w284:string)
            n96 = Bundle By Name(cluster=w275, "Core.Shutdown?"=TRUE) -> (w276:T5)
            n97 = call <vilib>:"Add State(s) to Queue__jki_lib_state_machine.vi"("State(s) in Front (\"\")"="Data: Cleanup\nEvents: Unregister", "State(s) in (\"\")"="Process: Sync", "State(s) at Back (\"\")"="Exit") -> ("States Out"=w279:string)  [unwired: 12 in]
            n98 = call <vilib>:"Add State(s) to Queue__jki_lib_state_machine.vi"("State(s) in (\"\")"=w284, "State(s) at Back (\"\")"=w279) -> ("States Out"=w283:string)  [unwired: 13 in]
            n99 = call <vilib>:"Add State(s) to Queue__jki_lib_state_machine.vi"("State(s) in Front (\"\")"=w283, "State(s) in (\"\")"=w289) -> ("States Out"=w288:string)  [unwired: 13 in]
          }
          frame "Macro: Post Error Handling" {
            # "Clear Last Error?"
            n100 = Unbundle By Name(w296) -> ("Core.Last Error.remaining states"=w298:string, "Core.Shutdown?"=w299:bool)
            n101 = Unbundle By Name(w296) -> ("Core.Last Error.error"=w291:errorcluster)
            n102 = case shown="False" FALSE {
              tunnel: w291 -> [w302 _]
              tunnel: [w302 _] -> w290
              frame False {
              }
              frame True {
              }
            }
            n103 = case shown="True" w299 {
              tunnel: w298 -> [w303 w305]
              tunnel: [w303 w304] -> w295
              frame False {
                # "These are the remaining states (at the moment the error occured). States can be altered according to business logic."
                # "NOT SHUTTING DOWN"
              }
              frame True {
                # "Developer can decide to alter the states but should be aware that during the shutdown process, there are certain states that must be run for the SMO to properly shut itself (and this process) down. As such, one can add states to perform additional clean-ups, but should append the remaining state to be executed."
                # "SHUTTING DOWN"
                n104 = call <vilib>:"Add State(s) to Queue__jki_lib_state_machine.vi"("State(s) in (\"\")"=w305) -> ("States Out"=w304:string)  [unwired: 14 in]
              }
            }
            n105 = Bundle By Name(cluster=w296, "Core.Last Error.error"=w290) -> (w297:T5)
            n106 = call <vilib>:"Add State(s) to Queue__jki_lib_state_machine.vi"("State(s) in Front (\"\")"=w295, "State(s) in (\"\")"=w293) -> ("States Out"=w294:string)  [unwired: 13 in]
          }
          frame "Macro: Debug" {
            # "exe?"
            # "If pane is an EXE, then close it when we exit"
            # "Macro: Debug\n(get debug behavior, determine UI and determine shutdown behavior)"
            n107 = Unbundle By Name(w309) -> ("Core.Close Panel on Exit?"=w312:bool, "SelfRef"=w317:refnum<class "Instrument.lvclass">)
            n108 = property class="App"() -> ("App.Kind"=w315:T1)  [unwired: 2 in, 2 out]
            n109 = Equal?(x=w315, y=T1."Run Time System" ("Application:Kind")) -> (x = y?=w311:bool)
            n110 = call <userlib>:"Get Debug Mode.vi"("error in (no error)"=w307, "SMO"=w317) -> ("error out"=w308:errorcluster, "Behavior"=w316:T9)  [unwired: 7 in, 1 out]
            n111 = case shown="\"Normal\", Default" w316 {
              tunnel: [w321 w323] -> w313
              tunnel: w312 -> [w321 _]
              tunnel: w311 -> [_ w325]
              tunnel: [_ "UI: Front Panel State >> Open\nUI: Wait >> 1000"] -> w306
              frame "Normal", Default {
                # "respect core.close"
              }
              frame "Debug" {
                # "keep panel open\nunless exe"
                n112 = Or(x=w325, y=FALSE) -> (x .or. y?=w323:bool)
              }
            }
            n113 = Bundle By Name(cluster=w309, "Core.Close Panel on Exit?"=w313) -> (w310:T5)
            n114 = call <vilib>:"Add State(s) to Queue__jki_lib_state_machine.vi"("State(s) in Front (\"\")"=w306, "State(s) in (\"\")"=w320) -> ("States Out"=w319:string)  [unwired: 13 in]
          }
          frame "---------- Process ----------" {
            # "Template Separator\n(You can make a copy of, or modify, this frame)"
            n115 = call <vilib>:"Add State(s) to Queue__jki_lib_state_machine.vi"("State(s) in (\"\")"=w330) -> ("States Out"=w329:string)  [unwired: 14 in]
          }
          frame "Process: Sync" {
            n116 = Unbundle By Name(w338) -> ("SelfRef"=w334:refnum<class "Instrument.lvclass">)
            n117 = call <vilib>:"WaitOnProcessSync.vi"("error in (no error)"=w333, "SMO"=w334) -> ("error out"=w332:errorcluster, "Don't run?"=w337:bool)  [unwired: 7 in, 1 out]
            n118 = Select(t="Data: Cleanup\nEvents: Unregister\nExit", s=w337, f="") -> (s? t:f=w331:string)
            n119 = call <vilib>:"Add State(s) to Queue__jki_lib_state_machine.vi"("State(s) in Front (\"\")"=w331, "State(s) in (\"\")"=w341) -> ("States Out"=w340:string)  [unwired: 13 in]
          }
          frame "Process: SelfTerminate" {
            # "Template Separator\n(You can make a copy of, or modify, this frame)"
            n120 = Unbundle By Name(w345) -> ("SelfRef"=w347:refnum<class "Instrument.lvclass">)
            n121 = call <vilib>:"SelfTerminate.vi"("error in (no error)"=w343, "SMO in"=w347) -> ("error out"=w342:errorcluster, "SMO out"=w346:refnum<class "Instrument.lvclass">)  [unwired: 8 in]
            n122 = Bundle By Name(cluster=w345, "SelfRef"=w346) -> (w344:T5)
            n123 = call <vilib>:"Add State(s) to Queue__jki_lib_state_machine.vi"("State(s) in (\"\")"=w350) -> ("States Out"=w349:string)  [unwired: 14 in]
          }
          frame "---------- Events ----------" {
            # "Template Separator\n(You can make a copy of, or modify, this frame)"
            n124 = call <vilib>:"Add State(s) to Queue__jki_lib_state_machine.vi"("State(s) in (\"\")"=w355) -> ("States Out"=w354:string)  [unwired: 14 in]
          }
          frame "Events: Register" {
            n125 = Unbundle By Name(w384) -> ("SelfRef"=w379:refnum<class "Instrument.lvclass">, "Dependencies.Remote-Control"=w378:refnum<class "RemoteControl.lvclass">, "Dependencies.DB-Logger"=w373:refnum<class "Logger.PGSQL.lvclass">, "Dependencies.Error-Logger"=w374:refnum<class "Logger.Error.lvclass">)
            n126 = call <vilib>:"GetProtectedEvents.vi"("SMO"=w379) -> ("error out"=w381:errorcluster, "SMO Protected Events"=w369:T10, "SMO out"=w372:refnum<class "Instrument.lvclass">)  [unwired: 8 in]
            n127 = call "Instrument.GetPrivateEvents.vi"("Instrument"=w372) -> ("error out"=w368:errorcluster, "Instrument Private Events"=w366:T11)  [unwired: 8 in, 1 out]
            n128 = call <userlib>:"RemoteControl.GetPublicEvents.vi"("RemoteControl"=w378) -> ("error out"=w367:errorcluster, "RC Public Events"=w365:T12, "RemoteControl out"=w371:refnum<class "RemoteControl.lvclass">)  [unwired: 8 in]
            n129 = call <vilib>:"GetPublicEvents.vi"("SMO"=w371) -> ("error out"=w377:errorcluster, "Public Events"=w364:T13)  [unwired: 8 in, 1 out]
            n130 = call <vilib>:"GetPublicEvents.vi"("SMO"=w373) -> ("error out"=w376:errorcluster, "Public Events"=w362:T13)  [unwired: 8 in, 1 out]
            n131 = call <vilib>:"GetPublicEvents.vi"("SMO"=w374) -> ("error out"=w375:errorcluster, "Public Events"=w359:T13)  [unwired: 8 in, 1 out]
            n132 = call "Rename RC SMO Private Events.vi"("error in (no error)"=w377, "Public Events"=w364) -> ("error out"=w356:errorcluster, "RC SMO Public Events"=w363:T13)  [unwired: 8 in]
            n133 = call "Rename PGSQL SMO Private Events.vi"("error in (no error)"=w376, "Public Events"=w362) -> ("error out"=w357:errorcluster, "PGSQL SMO Public Events"=w361:T13)  [unwired: 8 in]
            n134 = call "Rename Error SMO Private Events.vi"("error in (no error)"=w375, "Public Events"=w359) -> ("error out"=w360:errorcluster, "RC SMO Public Events"=w358:T13)  [unwired: 8 in]
            n135 = register-events(w369, w366, w365, w363, w361, w358) -> (reference out=w383:refnum<event-registration>, error out=w370:errorcluster)  [unwired: 2 in]
            n136 = Merge Errors(w370, w356, w357, w360, w367, w368, w381, w380) -> (w382:errorcluster)
            n137 = call <vilib>:"Add State(s) to Queue__jki_lib_state_machine.vi"("State(s) in (\"\")"=w386) -> ("States Out"=w385:string)  [unwired: 14 in]
          }
          frame "Events: Unregister" {
            n138 = Unregister For Events(event registration refnum=w389, error in=w388) -> (error out=w387:errorcluster)
            n139 = call <vilib>:"Clear Errors.vi"("error in (no error)"=w387) -> ()  [unwired: 5 in, 2 out]
            n140 = call <vilib>:"Add State(s) to Queue__jki_lib_state_machine.vi"("State(s) in (\"\")"=w392) -> ("States Out"=w391:string)  [unwired: 14 in]
          }
          frame "---------- Instrument ----------" {
            n141 = call <vilib>:"Add State(s) to Queue__jki_lib_state_machine.vi"("State(s) in (\"\")"=w397) -> ("States Out"=w396:string)  [unwired: 14 in]
          }
          frame "Instrument: Handle Command" {
            # "parse and handle incoming commands\n- respond with data on hand\n- forward message to child instrument...etc"
            n142 = Unbundle By Name(w413) -> ("Dependencies.Remote-Control"=w417:refnum<class "RemoteControl.lvclass">, "SelfRef"=w414:refnum<class "Instrument.lvclass">, "Message.Command"=w398:string, "Message.Data"=w411:variant, "Message.ID"=w415:string)
            n143 = Format Into String(format string="%s Command:  %s", w400, w398) -> (resulting string=→"Command":string)  [unwired: 2 in, 1 out]
            n144 = call-dynamic "Handle Command.vi"("error in (no error)"=w416, "params in"=w411, "command"=w398, "Instrument in"=w414) -> ("error out"=w404:errorcluster, "processed data"=w407:variant, "command out"=w406:string, "Instrument out"=w403:refnum<class "Instrument.lvclass">)  [unwired: 4 in]
            n145 = Empty String/Path?(string/path=w406) -> (empty?=w410:bool)
            n146 = Empty String/Path?(string/path=w407) -> (empty?=w409:bool)
            n147 = And(x=w410, y=w409) -> (x .and. y?=w408:bool)
            n148 = case shown="False" w408 {
              tunnel: w417 -> [w429 _]
              tunnel: w404 -> [w425 w447]
              tunnel: w407 -> [w427 _]
              tunnel: w415 -> [w428 _]
              tunnel: [w424 w447] -> w405
              tunnel: w406 -> [w426 _]
              tunnel: w400 -> [w423 _]
              tunnel: w403 -> [w422 w446]
              tunnel: [w421 w446] -> w402
              frame False {
                # "command respond"
                n149 = case shown="\"Remote\"" w423 {
                  tunnel: w429 -> [_ w445]
                  tunnel: w428 -> [w431 w438]
                  tunnel: w427 -> [w433 w437]
                  tunnel: w426 -> [w434 w439]
                  tunnel: w425 -> [w432 w444]
                  tunnel: [w430 w443] -> w424
                  tunnel: w422 -> [w436 w440]
                  tunnel: [w435 w440] -> w421
                  frame "Local", Default {
                    n150 = call "Instrument.sendMessageFromProcess.vi"("ID"=w431, "error in (no error)"=w432, "Data"=w433, "Command"=w434, "Instrument"=w436) -> ("error out"=w430:errorcluster, "Instrument out"=w435:refnum<class "Instrument.lvclass">)  [unwired: 5 in]
                  }
                  frame "Remote" {
                    n151 = Bundle By Name(cluster=T3 {"Command"="", "Data"=variant(string ""), "ID"=""} ("Message"), "Command"=w439, "Data"=w437, "ID"=w438) -> (w441:T3)
                    n152 = call <userlib>:"RemoteControl.SendMessageToProcess.vi"("error in (no error)"=w444, "Message"=w441, "RemoteControl"=w445) -> ("error out"=w443:errorcluster)  [unwired: 7 in, 1 out]
                  }
                }
              }
              frame True {
              }
            }
            n153 = Bundle By Name(cluster=w413, "SelfRef"=w402) -> (w412:T5)
            n154 = call <vilib>:"Add State(s) to Queue__jki_lib_state_machine.vi"("State(s) in (\"\")"=w420) -> ("States Out"=w419:string)  [unwired: 14 in]
          }
        }
      }
    }
    frame Error {
    }
  }
  n155 = call-parent "Process.vi"("error in"=w5, "SMO"=w4) -> ("error out"=w2:errorcluster, "SMO out"=→"Instrument out":refnum<class "Instrument.lvclass">)  [unwired: 8 in]
  n156 = Merge Errors(w2, w1) -> (→"error out":errorcluster)
